vi "myRIO_BRig_RT_dataLC_ENL1_Probability_Switch_l2.vi"() -> (2 "output_ENL1_Probability_Switch_l2":i32)   [LabVIEW 2014]
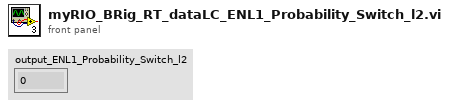
[diagram p1: front panel]
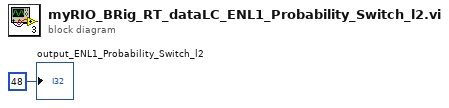
[diagram p0: block diagram]
diagram:
  "output_ENL1_Probability_Switch_l2" <- 48 ("output_iBlock")
